vi "split_hist11.vi"(2 "N":i32, 3 "hist in":cluster{"values":i16[], "q":i32[]}) -> (0 "remainder hist":cluster{"values":i16[], "q":i32[]}, 1 "first N valued hist":cluster{i16[], i32[]})   [LabVIEW 2010]
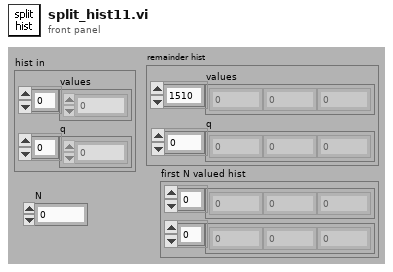
[diagram p1: front panel]
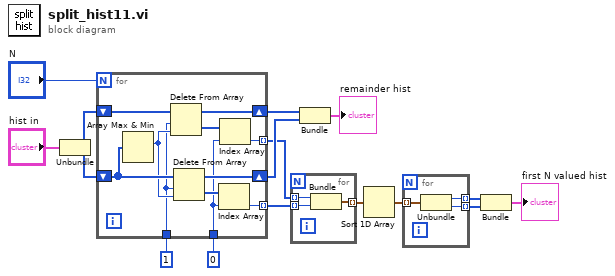
[diagram p0: block diagram]
diagram:
  n1 = Unbundle("hist in") -> ("values"=w13:i16[], "q"=w14:i32[])
  n2 = for {
    N: "N" -> [_]
    shift-right: [w26] -> w11
    shift-left: w13 -> [w27]
    shift-right: [w24] -> w10
    shift-left: w14 -> [w25]
    tunnel: 1 -> [w22]
    tunnel: [w20] -> w8 mode=indexing
    tunnel: [w18] -> w9 mode=indexing
    tunnel: 0 -> [w17]
    n3 = Array Max & Min(array=w25) -> (max index (indices)=w23:i32)  [unwired: 3 out]
    n4 = Delete From Array(array=w27, length=w22, index=w23) -> (deleted portion=w21:i16[], array with subset deleted=w26:i16[])
    n5 = Delete From Array(array=w25, length=w22, index=w23) -> (deleted portion=w19:i32[], array with subset deleted=w24:i32[])
    n6 = Index Array(array=w19, index=w17) -> (element=w18:i32)
    n7 = Index Array(array=w21, index=w17) -> (element=w20:i16)
  }
  n8 = for {
    tunnel: w9 -> [w30] mode=indexing
    tunnel: w8 -> [w29] mode=indexing
    tunnel: [w28] -> w5 mode=indexing
    n9 = Bundle(w29, "element"=w30) -> (w28:cluster{i16, "element":i32})  [unwired: 1 in]
  }
  n10 = Bundle("values"=w11, "q"=w10) -> (→"remainder hist":cluster{"values":i16[], "q":i32[]})  [unwired: 1 in]
  n11 = Sort 1D Array(array=w5) -> (sorted array=w4:cluster{i16, "element":i32}[])
  n12 = for {
    tunnel: w4 -> [w33] mode=indexing
    tunnel: [w32] -> w2 mode=indexing
    tunnel: [w31] -> w3 mode=indexing
    n13 = Unbundle(w33) -> (w32:i16, "element"=w31:i32)
  }
  n14 = Bundle(w2, w3) -> (→"first N valued hist":cluster{i16[], i32[]})  [unwired: 1 in]
